vi "FourFlippingCoins.vi"() -> ()   [LabVIEW 2014]
panel:
  in  "Number of trails":dbl
  out "Waveform Graph":dynamicdata(graph)
  out "Number of Heads":dbl
  out "Coin 4":bool
  out "Coin 3":bool
  out "Coin 2":bool
  out "Coin 1":bool
  # "Heads = Lit"
  # "Tails = Unlit"
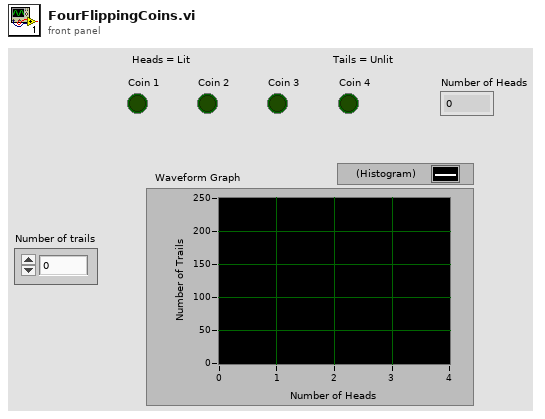
[diagram p1: front panel]
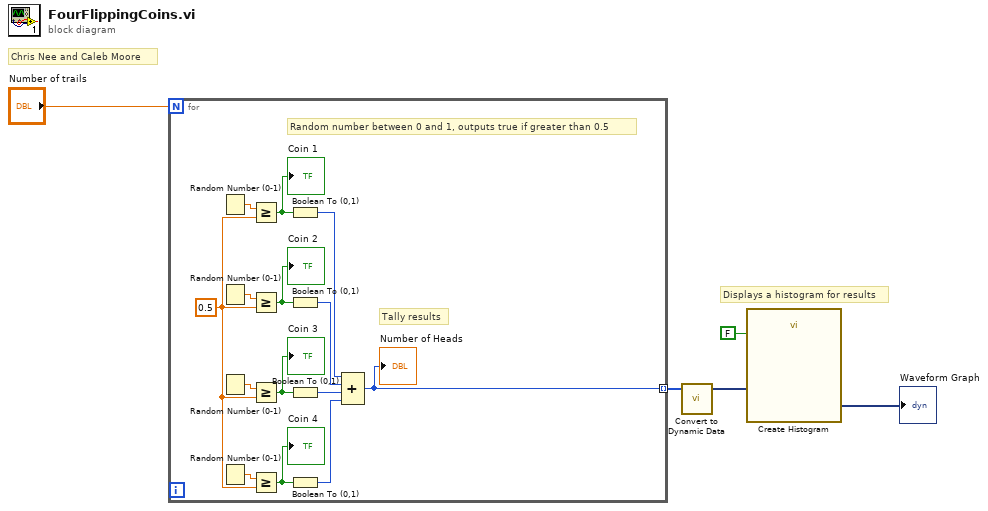
[diagram p0: block diagram]
diagram:
  # "Chris Nee and Caleb Moore"
  # "Displays a histogram for results"
  n1 = for {
    N: "Number of trails" -> [_]
    tunnel: [w6] -> w3 mode=indexing
    w16 = 0.5
    # "Tally results"
    # "Random number between 0 and 1, outputs true if greater than 0.5"
    n2 = Random Number (0-1)() -> (number: 0 to 1=w19:dbl)
    n3 = Random Number (0-1)() -> (number: 0 to 1=w15:dbl)
    n4 = Random Number (0-1)() -> (number: 0 to 1=w14:dbl)
    n5 = Random Number (0-1)() -> (number: 0 to 1=w13:dbl)
    n6 = Greater Or Equal?(x=w19, y=w16) -> (x >= y?=w18:bool)
    "Coin 1" <- w18
    n7 = Greater Or Equal?(x=w15, y=w16) -> (x >= y?=w12:bool)
    "Coin 2" <- w12
    n8 = Greater Or Equal?(x=w14, y=w16) -> (x >= y?=w11:bool)
    "Coin 3" <- w11
    n9 = Greater Or Equal?(x=w13, y=w16) -> (x >= y?=w10:bool)
    "Coin 4" <- w10
    n10 = Boolean To (0,1)(Boolean=w18) -> (0, 1=w17:i16)
    n11 = Boolean To (0,1)(Boolean=w12) -> (0, 1=w9:i16)
    n12 = Boolean To (0,1)(Boolean=w11) -> (0, 1=w8:i16)
    n13 = Boolean To (0,1)(Boolean=w10) -> (0, 1=w7:i16)
    n14 = Compound Arithmetic op=ADD(w17, w9, w8, w7) -> (w6:i16)
    "Number of Heads" <- w6
  }
  n15 = call "Convert to Dynamic Data"("Array"=w3) -> ("Dynamic Data Type"=w2:dynamicdata)  [unwired: 3 in]
  n16 = call "Create Histogram"("Reset"=FALSE, "Signal"=w2) -> ("Histogram"=→"Waveform Graph":dynamicdata)  [unwired: 8 in, 1 out]
